vi "AutoMatch.vi"() -> ()   [LabVIEW 2018]
panel:
  out "Number of Iterations":i32
  out "Current Number":u32 format="%#.0f"
  in  "Number to Match":u32=50 max=1000 step=1
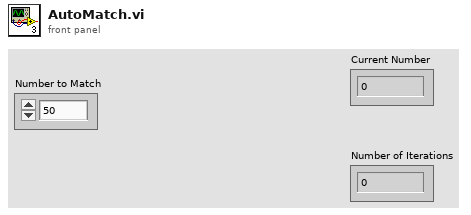
[diagram p1: front panel]
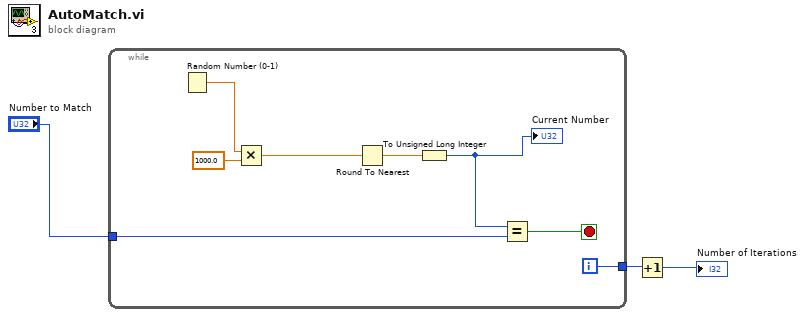
[diagram p0: block diagram]
diagram:
  n1 = while {
    tunnel: [w8] -> w3
    tunnel: "Number to Match" -> [w5]
    i -> [w8]
    stop <- w9 stop-if-true
    n2 = Random Number (0-1)() -> (number: 0 to 1=w10:dbl)
    n3 = Multiply(x=w10, y=1000.0) -> (x*y=w7:dbl)
    n4 = Round To Nearest(number=w7) -> (nearest integer value=w6:dbl)
    n5 = To Unsigned Long Integer(number=w6) -> (unsigned 32bit integer=w4:u32)
    "Current Number" <- w4
    n6 = Equal?(x=w4, y=w5) -> (x = y?=w9:bool)
  }
  n7 = Increment(x=w3) -> (x+1=→"Number of Iterations":i32)
